vi "ConnectSetPVs.vi"(8 "error in (no error)":errorcluster, 10 "Set-Messages":string[](array[string]), 11 "CS++GUIActor in":refnum<class "CS++GUIActor.lvclass">) -> (0 "error out":errorcluster, 2 "PVConnections":refnum<class "PVConnection.lvclass">[](array[class]), 3 "CS++GUIActor out":refnum<class "CS++GUIActor.lvclass">)   [LabVIEW 2014, in "CS++GUIActor.lvlib" / "CS++GUIActor.lvclass"]
doc: "Opens the connection to (already existing) PVs to set values."
uses:
  CS++GUIActor.lvclass
  Classes/CS++ProcessVariables/PVConnection/PVConnection.lvclass
  CS++BaseActor/CS++BaseActor.lvclass/CS++BaseActor.ctl
  CS++GUIActor.lvclass/CS++GUIActor.ctl
  Classes/CS++ProcessVariables/ProcessVariable/PV.lvclass
  Classes/CS++ProcessVariables/ProcessVariable/PV.lvclass/PV.ctl
  Classes/CS++ProcessVariables/ProcessVariable/Write Name.vi
  Classes/CS++ProcessVariables/ProcessVariable/Write PV URL.vi
  CS++BaseActor/Read CS++Factory.vi
  Read Associated Proxy Actor Name.vi
  Classes/CS++BaseClasses/Factory/CS++Factory.lvclass
  Classes/CS++ProcessVariables/CS++ProcessVariables.lvlib
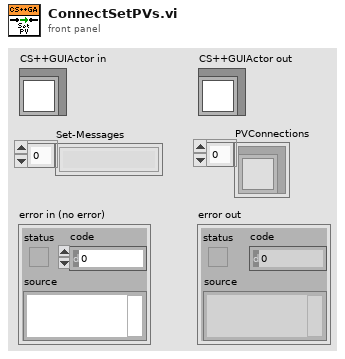
[diagram p1: front panel]
types:
  T1 = cluster{"Read Access":enum8{"Allowed", "Required", "None"}, "Write Access":enum8{"Allowed", "Required", "None"}}
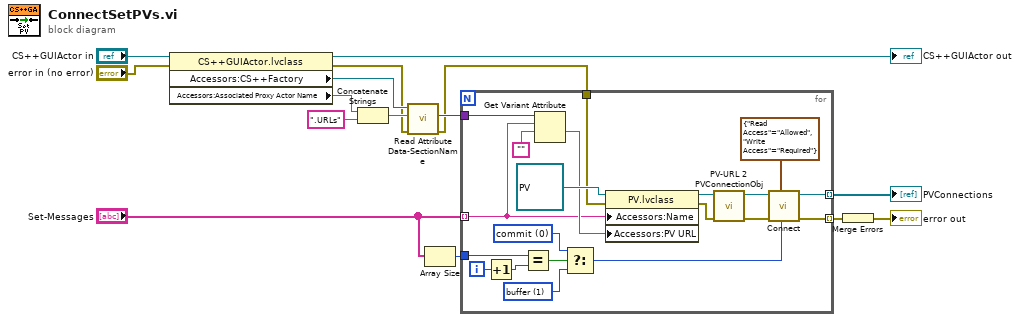
[diagram p0: block diagram]
diagram:
  n1 = property class="CS++GUIActor.lvclass"(reference="CS++GUIActor in", error in="error in (no error)") -> (reference out=→"CS++GUIActor out":refnum<class "CS++GUIActor.lvclass">, error out=w3:errorcluster, "Accessors:CS++Factory"=w8:refnum<class "CS++Factory.lvclass">, "Accessors:Associated Proxy Actor Name"=w10:string)
  n2 = Concatenate Strings(w10, ".URLs" ("Object Name")) -> (w9:string)
  n3 = call-dynamic "Read Attribute Data-SectionName.vi"("error in (no error)"=w3, "Object Name"=w9, "CS++Factory in"=w8) -> ("error out"=w2:errorcluster, "Attribute Data"=w12:variant)  [unwired: 6 in, 1 out]
  n4 = Array Size(array="Set-Messages") -> (size(s)=w7:i32)
  n5 = for {
    tunnel: w2 -> [w29]
    tunnel: w12 -> [w28]
    tunnel: "Set-Messages" -> [w25] mode=indexing
    tunnel: w7 -> [w23]
    tunnel: [w17] -> w6 mode=indexing
    tunnel: [w16] -> w5 mode=indexing
    i -> [w24]
    w20 = u16 0 items=["commit", "buffer"] ("Mode (buffer)")
    w19 = u16 1 items=["commit", "buffer"] ("Mode (buffer)")
    n6 = Increment(x=w24) -> (x+1=w22:i32)
    n7 = Equal?(x=w23, y=w22) -> (x = y?=w21:bool)
    n8 = Get Variant Attribute(Variant=w28, name=w25, default value (empty Variant)="") -> (value=w26:string)  [unwired: 1 in, 3 out]
    n9 = Select(t=w20, s=w21, f=w19) -> (s? t:f=w18:u16)
    n10 = property class="PV.lvclass"(reference=refnum<class "PV.lvclass"> refnum ("CS++ProcessVariables.lvlib:PV.lvclass"), error in=w29, "Accessors:Name"=w25, "Accessors:PV URL"=w26) -> (reference out=w33:refnum<class "PV.lvclass">, error out=w31:errorcluster)
    n11 = call "PV-URL 2 PVConnectionObj.vi"("Error In"=w31, "PV"=w33) -> ("Error Out"=w35:errorcluster, "PVConnection"=w34:refnum<class "PVConnection.lvclass">)  [unwired: 7 in, 1 out]
    n12 = call "Connect.vi"("Access (R/W allowed)"=T1 {"Read Access"=enum."Allowed", "Write Access"=enum."Required"}, "Mode (buffer)"=w18, "Error In"=w35, "PVConnection in"=w34) -> ("Error Out"=w16:errorcluster, "PVConnection out"=w17:refnum<class "PVConnection.lvclass">)  [unwired: 6 in]
  }
  "PVConnections" <- w6
  n13 = Merge Errors(w5) -> (→"error out":errorcluster)
